vi "test dopasowania skal1.vi"() -> ()   [LabVIEW 2014]
panel:
  out "skala wy":i32
  out "Zakresy wy":cluster{"Zakresy":dbl[], "skale":i32[]}
  in  "szukany zakres 2":dbl
  in  "Zakresy we":cluster{"Zakresy":dbl[], "skale":i32[]}
  out "element 2":i32
  in  "szukany zakres":dbl
  in  "Zakresy":cluster{"Zakresy":dbl[], "skale":i32[]}
  out "index of element":i32
  in  "element":cluster{"Zakres":dbl, "skala":i32}
  in  "Array":cluster{"Zakres":dbl, "skala":i32}[](array[cluster])
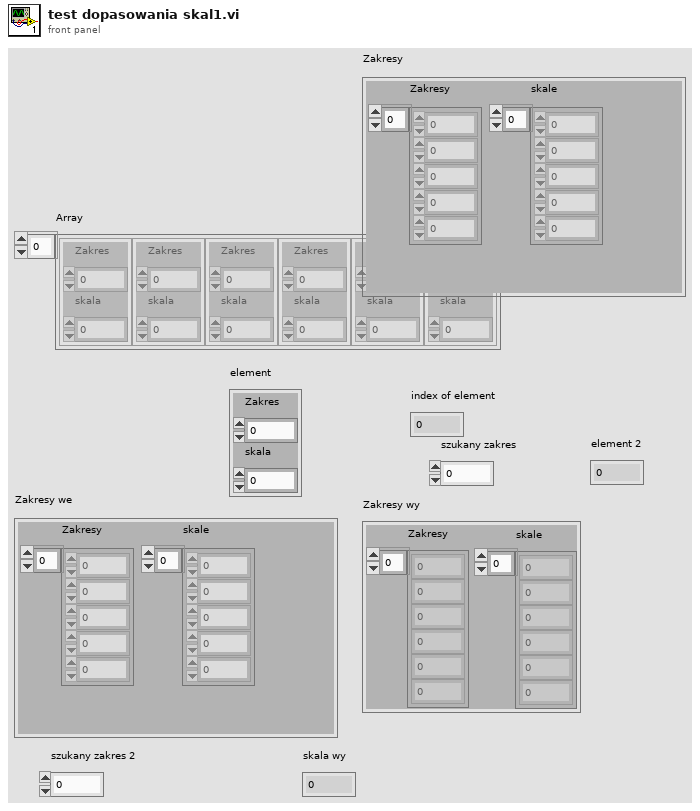
[diagram p1: front panel]
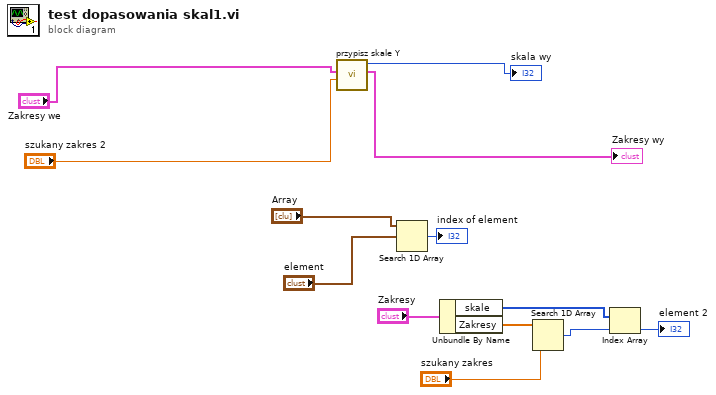
[diagram p0: block diagram]
diagram:
  n1 = call "przypisz skale Y.vi"("szukany zakres in"="szukany zakres 2", "Zakresy we"="Zakresy we") -> ("Zakresy wy"=→"Zakresy wy":cluster{"Zakresy":dbl[], "skale":i32[]}, "skala wy"=→"skala wy":i32)  [unwired: 7 in, 1 out]
  n2 = Search 1D Array(1D array="Array", element="element") -> (index of element=→"index of element":i32)  [unwired: 1 in]
  n3 = Unbundle By Name("Zakresy") -> ("skale"=w6:i32[], "Zakresy"=w9:dbl[])
  n4 = Search 1D Array(1D array=w9, element="szukany zakres") -> (index of element=w7:i32)  [unwired: 1 in]
  n5 = Index Array(array=w6, index=w7) -> (element=→"element 2":i32)
